vi "SMU.TestLauncher.vi"() -> ()   [LabVIEW 2017, in "SMU.lvclass"]
doc: "JKI State Machine Objects (SMO) 1.0.0.5\nJKI - JKI\nCopyright (c) 2016, JKI"
uses:
  SMU.lvclass
  <vilib>/JKI/JKI SMO/SMO/Typedefs/SMOState --Enum.ctl
  SMU.Keithley2600/SMU.Keithley2600.lvclass
  SMU.Simulated/SMU.Simulated.lvclass
  D:/upwork/Laser Measurement Tool/Laser/project/Subsystems/SMU/SMU.lvclass
  D:/Program Files (x86)/National Instruments/LabVIEW 2017/vi.lib/JKI/JKI SMO/SMO/SMO.lvclass
  D:/upwork/Laser Measurement Tool/Laser/project/Subsystems/MeasuringDevice/MeasuringDevice.lvclass
  <vilib>/JKI/JKI SMO/SMO/SMO.lvclass
  MeasuringDevice/MeasuringDevice.lvclass
panel:
  out "Current Measurements":dbl[](array[numeric])
  out "Current, A":dbl
  in  "Measure":bool
  out "SMO State":T1
  out "error out":errorcluster
  in  "Stop":bool
  # "SMU Test Launcher"
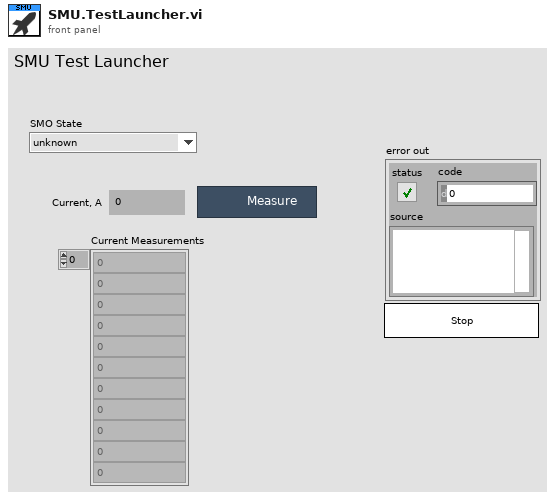
[diagram p1: front panel]
types:
  T1 = typedef "SMO.lvclass/SMOState --Enum.ctl" = enum16{"unknown", "Created", "Started", "Stopped"}
  T2 = typedef "MeasuringDevice.lvclass/PublicEvents--Cluster.ctl" = cluster{"MeasurementCompleted":refnum<user-event>}
  T3 = typedef "SMO.lvclass/Public Events.ctl" = cluster{"Error":refnum<user-event>, "State":refnum<user-event>, "Reserve State":refnum<user-event>}
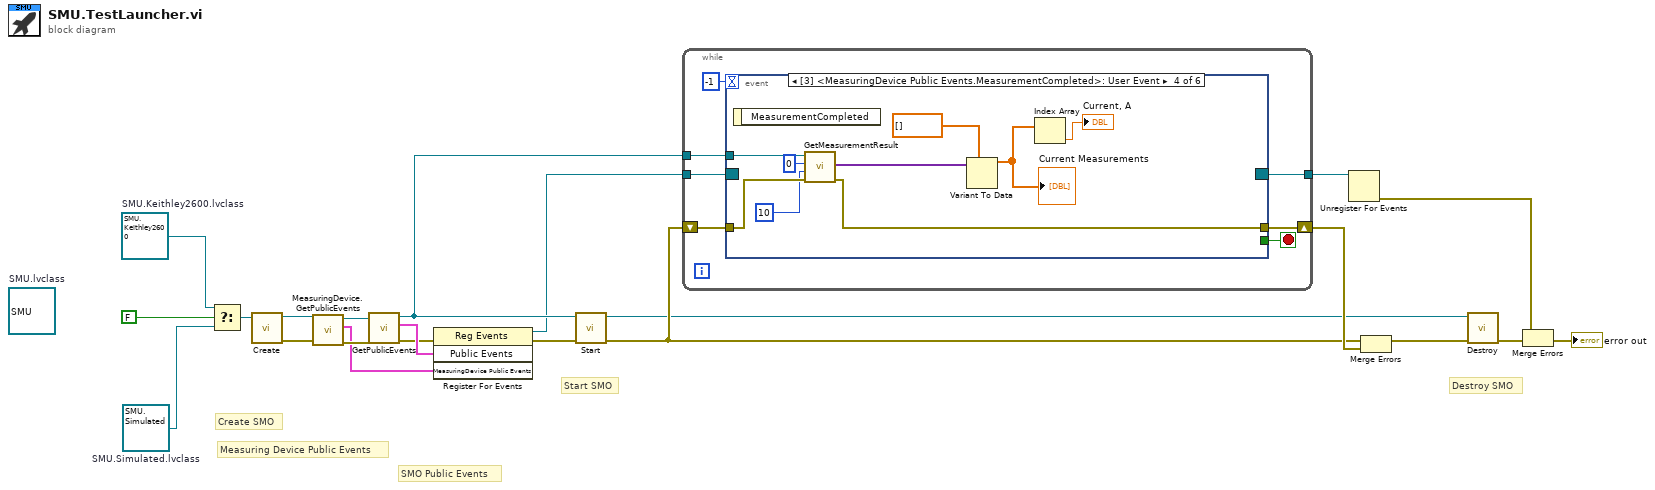
[diagram p0: block diagram]
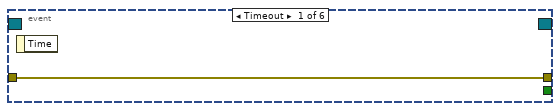
[diagram p2: hidden frame]
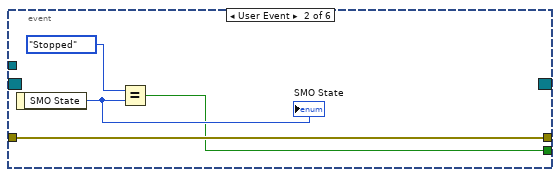
[diagram p3: hidden frame]
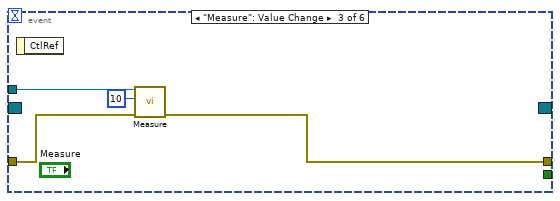
[diagram p4: hidden frame]
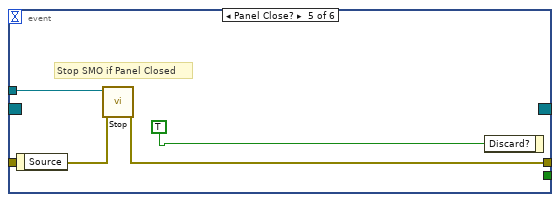
[diagram p5: hidden frame]
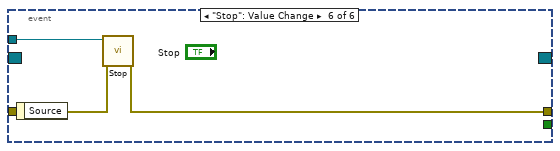
[diagram p6: hidden frame]
diagram:
  (unwired) refnum<class "SMU.lvclass"> refnum  # SMU.lvclass
  w1 = refnum<class "SMU.Simulated.lvclass"> refnum  # SMU.Simulated.lvclass
  w9 = refnum<class "SMU.Keithley2600.lvclass"> refnum  # SMU.Keithley2600.lvclass
  # "Measuring Device Public Events"
  # "SMO Public Events"
  # "Start SMO"
  # "Destroy SMO"
  # "Create SMO"
  n1 = Select(t=w9, s=FALSE, f=w1) -> (s? t:f=w8:refnum<class "SMU.lvclass">)
  n2 = call <vilib>:"Create.vi"("SMO"=w8) -> ("error out"=w5:errorcluster, "SMO out"=w6:refnum<class "SMU.lvclass">)  [unwired: 8 in, 1 out]
  n3 = call "MeasuringDevice.GetPublicEvents.vi"("error in (no error)"=w5, "MeasuringDevice"=w6) -> ("error out"=w4:errorcluster, "MeasuringDevice Public Events"=w2:T2, "MeasuringDevice out"=w3:refnum<class "SMU.lvclass">)  [unwired: 7 in]
  n4 = call <vilib>:"GetPublicEvents.vi"("error in (no error)"=w4, "SMO"=w3) -> ("error out"=w11:errorcluster, "Public Events"=w12:T3, "SMO out"=w14:refnum<class "SMU.lvclass">)  [unwired: 7 in]
  n5 = register-events(error in=w11, w12, w2) -> (reference out=w10:refnum<event-registration>, error out=w13:errorcluster)  [unwired: 1 in]
  n6 = call <vilib>:"Start.vi"("error in (no error)"=w13, "SMO"=w14) -> ("error out"=w17:errorcluster, "SMO out"=w15:refnum<class "SMU.lvclass">)  [unwired: 8 in]
  n7 = while {
    shift-right: [w28] -> w21
    shift-left: w17 -> [w27]
    tunnel: w10 -> [w26]
    tunnel: [w25] -> w22
    tunnel: w14 -> [w24]
    stop <- w29 stop-if-true
    n8 = event shown="[3] <MeasuringDevice Public Events.MeasurementCompleted>: User Event" {
      selector: w26 -> [_ _ _ _ _ _]
      dyn-events: [_ _ _ _ _ _] -> w25
      timeout: -1 -> [_ _ _ _ _ _]
      tunnel: [_ w31 _ _ _ _] -> w29
      tunnel: w24 -> [_ _ w38 w47 w51 w54]
      tunnel: [w30 w34 w36 w45 w50 w53] -> w28
      tunnel: w27 -> [w30 w34 w37 w46 w49 w52]
      event Timeout {
        n9 = event-data() -> ()  [unwired: 1 in, 1 out]
      }
      event User Event {
        n10 = event-data() -> ("SMO State"=w33:T1)  [unwired: 1 in]
        "SMO State" <- w33
        n11 = Equal?(x=SMOState_--Enum."Stopped", y=w33) -> (x = y?=w31:bool)
      }
      event "Measure": Value Change {
        n12 = event-data() -> ()  [unwired: 1 in, 1 out]
        n13 = call "Measure.vi"("error in (no error)"=w37, "Count (1)"=u16 10, "MeasuringDevice"=w38) -> ("error out"=w36:errorcluster)  [unwired: 6 in, 2 out]
      }
      event User Event {
        n14 = event-data() -> ()  [unwired: 1 in, 1 out]
        n15 = call "GetMeasurementResult.vi"("error in (no error)"=w46, "Count (1)"=10, "Offset (0)"=0, "MeasuringDevice in"=w47) -> ("error out"=w45:errorcluster, "Result"=w43:variant[])  [unwired: 5 in, 1 out]
        n16 = Variant To Data(type=dbl[] [], Variant=w43) -> (data=w42:dbl[])  [unwired: 1 in, 1 out]
        "Current Measurements" <- w42
        n17 = Index Array(array=w42) -> (element=→"Current, A":dbl)  [unwired: 1 in]
      }
      event Panel Close? {
        # "Stop SMO if Panel Closed"
        n18 = event-data() -> ()  [unwired: 1 in, 1 out]
        n19 = call <vilib>:"Stop.vi"("error in (no error)"=w49, "SMO"=w51) -> ("error out"=w50:errorcluster)  [unwired: 8 in, 1 out]
        n20 = event-data("Discard?"=TRUE ("OK")) -> ()  [unwired: 1 in, 1 out]
      }
      event "Stop": Value Change {
        n21 = event-data() -> ()  [unwired: 1 in, 1 out]
        n22 = call <vilib>:"Stop.vi"("error in (no error)"=w52, "SMO"=w54) -> ("error out"=w53:errorcluster)  [unwired: 8 in, 1 out]
      }
    }
  }
  n23 = Unregister For Events(event registration refnum=w22) -> (error out=w20:errorcluster)  [unwired: 1 in]
  n24 = Merge Errors(w17, w21) -> (w16:errorcluster)
  n25 = call <vilib>:"Destroy.vi"("error in (no error)"=w16, "SMO"=w15) -> ("error out"=w18:errorcluster)  [unwired: 9 in]
  n26 = Merge Errors(w20, w18) -> (→"error out":errorcluster)
